vi "Query Output Operation State.vi"(0 "VISA resource name":refnum<visa-resource-name>, 11 "error in (no error)":errorcluster) -> (2 "Voltage Setpoint (V)":dbl format="%#.6g", 3 "Current Setpoint (A)":dbl format="%#.6g", 4 "VISA resource name out":refnum<visa-resource-name>, 6 "Mode (0: Off)":i32(ring) items=["Off", "Standby", "Charge", "Discharge", "Battery"], 8 "Enable":T1, 13 "Power Setpoint (W)":dbl format="%#.6g", 14 "Resistance Setpoint (Ohms)":dbl format="%#.6g", 15 "error out":errorcluster)   [LabVIEW 2012, in "NH Research Regenerative Test Series.lvlib"]
doc: "Query the present operation mode and settings."
uses:
  <instrlib>/NH Research Regenerative Test Series/NH Research Regenerative Test Series.lvlib
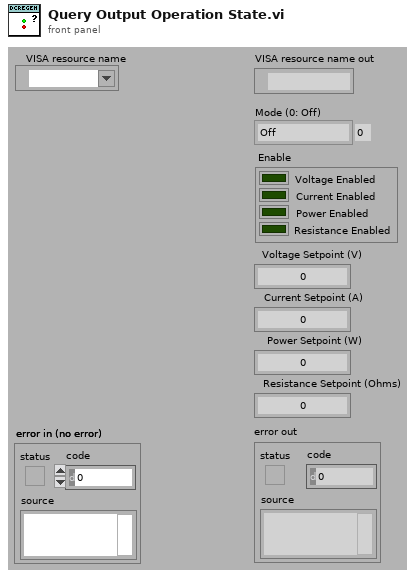
[diagram p1: front panel]
types:
  T1 = cluster{"Voltage Enabled":bool, "Current Enabled":bool, "Power Enabled":bool, "Resistance Enabled":bool}
  T2 = cluster{"Boolean array[0]":bool, "Boolean array[1]":bool, "Boolean array[2]":bool, "Boolean array[3]":bool}
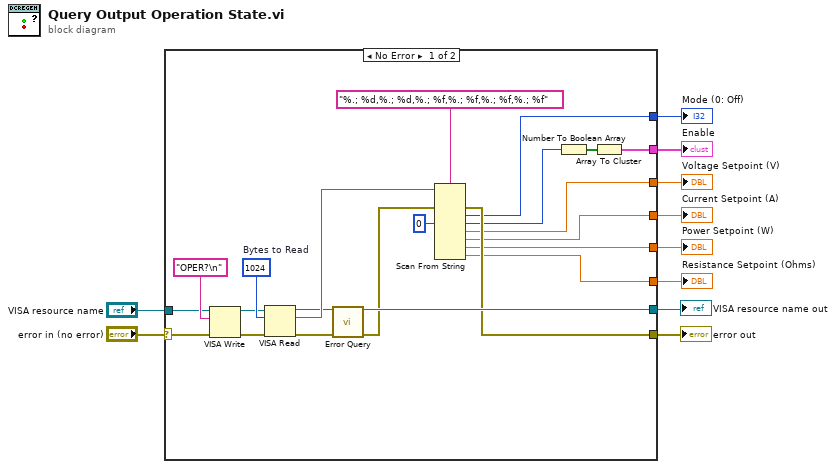
[diagram p0: block diagram]
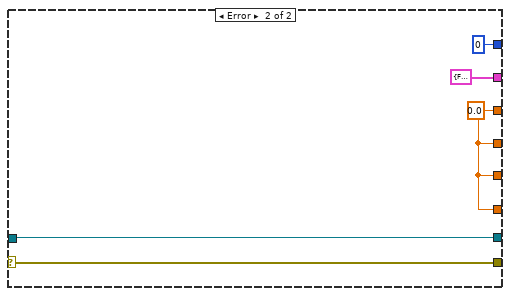
[diagram p2: hidden frame]
diagram:
  n1 = case shown="No Error" "error in (no error)" {
    selector: "error in (no error)" -> [w28 w37]
    tunnel: [w20 w37] -> w9
    tunnel: [w24 w36] -> w7
    tunnel: "VISA resource name" -> [w27 w36]
    tunnel: [w19 0] -> w6
    tunnel: [w15 T2 {"Boolean array[0]"=FALSE, "Boolean array[1]"=FALSE, "Boolean array[2]"=FALSE, "Boolean array[3]"=FALSE} ("Boolean array")] -> w5
    tunnel: [w14 w33] -> w4
    tunnel: [w13 w33] -> w3
    tunnel: [w12 w33] -> w2
    tunnel: [w11 w33] -> w1
    frame No Error {
      w32 = u32 1024  # Bytes to Read
      n2 = VISA Write(VISA resource name=w27, write buffer="OPER?\n", error in (no error)=w28) -> (VISA resource name out=w30:refnum<visa-resource-name>, error out=w31:errorcluster)  [unwired: 1 out]
      n3 = VISA Read(VISA resource name=w30, byte count=w32, error in (no error)=w31) -> (VISA resource name out=w23:refnum<visa-resource-name>, read buffer=w26:string, error out=w22:errorcluster)  [unwired: 1 out]
      n4 = call <instrlib>:"Error Query.vi"("VISA resource name"=w23, "error in (no error)"=w22) -> ("VISA resource name out"=w24:refnum<visa-resource-name>, "error out"=w21:errorcluster)  [unwired: 10 in, 2 out]
      n5 = Scan From String(format string="%.; %d,%.; %d,%.; %f,%.; %f,%.; %f,%.; %f", input string=w26, error in=w21, default 2=u8 0 ("default value 2")) -> (error out=w20:errorcluster, output 1=w19:i32, output 2=w16:u8, output 3=w14:dbl, output 4=w13:dbl, output 5=w12:dbl, output 6=w11:dbl)  [unwired: 6 in, 2 out]
      n6 = Number To Boolean Array(number=w16) -> (Boolean array=w18:bool[])
      n7 = Array To Cluster(array=w18) -> (cluster=w15:T2)
    }
    frame Error {
      w33 = 0.0
    }
  }
  "error out" <- w9
  "VISA resource name out" <- w7
  "Power Setpoint (W)" <- w2
  "Enable" <- w5
  "Voltage Setpoint (V)" <- w4
  "Current Setpoint (A)" <- w3
  "Resistance Setpoint (Ohms)" <- w1
  "Mode (0: Off)" <- w6
